vi "SN_regular_expression_based_parser.vi"(7 "regular expression":string, 8 "error in (no error)":errorcluster, 11 "SN in":string) -> (0 "error out":errorcluster, 1 "SN status":enum16{"SN PASS", "SN FAIL"}(ring), 2 "match?":bool, 3 "SN out":string)   [LabVIEW 2024]
panel:
  # "<-- Lit when match"
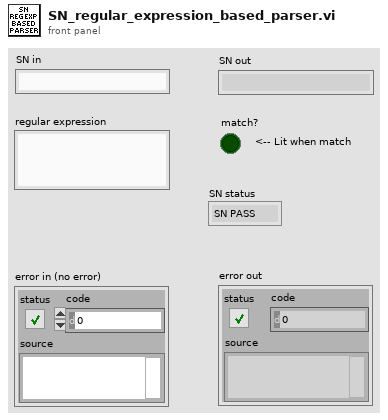
[diagram p1: front panel]
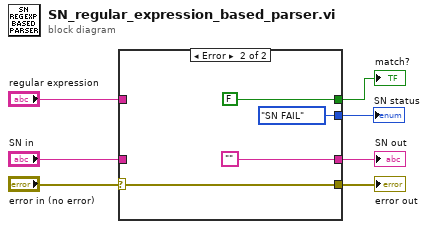
[diagram p0: block diagram]
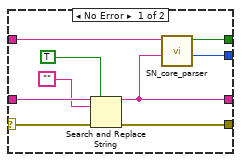
[diagram p2: hidden frame]
diagram:
  n1 = case shown="Error" "error in (no error)" {
    selector: "error in (no error)" -> [w15 w20]
    tunnel: [w14 w20] -> w6
    tunnel: "SN in" -> [w13 _]
    tunnel: [w10 ""] -> w4
    tunnel: [w11 FALSE] -> w3
    tunnel: "regular expression" -> [w9 _]
    tunnel: [w8 enum16{"SN PASS", "SN FAIL"}."SN FAIL" ("SN status")] -> w1
    frame No Error {
      n2 = Search and Replace String(replace all?=TRUE ("replace all? (F)"), input string=w13, search string="", error in=w15) -> (result string=w10:string, error out=w14:errorcluster)  [unwired: 4 in, 2 out]
      n3 = call "SN_core_parser.vi"("SN in"=w10, "regular expression"=w9) -> ("SN status"=w8:enum16{"SN PASS", "SN FAIL"}, "match?"=w11:bool)  [unwired: 8 in]
    }
    frame Error {
    }
  }
  "error out" <- w6
  "SN out" <- w4
  "match?" <- w3
  "SN status" <- w1
